vi "GUI.Config Test GENERICO.vi"() -> ()   [LabVIEW 2009]
panel:
  in  "QUIT 2":bool
  in  "QUIT":bool
  in  "default":bool
  in  "Limits Measurements ADC":string[][](table)
  in  "stop":bool
  in  "Lim offset Dig":cluster{"Max Dig":dbl}={"Max Dig"=0.05} {"Max Dig" format="%.3g"}
  in  "Lim Offset Analog":cluster{"Max Analog":dbl, "Min Analog":dbl}={"Max Analog"=0.05, "Min Analog"=-0.05} {"Min Analog" format="%.3g"; "Max Analog" format="%.3g"}
  in  "Vin Rate Adders":i32[](listbox)
  in  "Limits Rate Scan":cluster{"High":dbl[], "Low":dbl[]}={"High"=[0.15, 0.242, 0.331, 0.425, 0.512, 0.6, 0.688, 0.774, 0.847, 0.91], "Low"=[0.021, 0.11, 0.189, 0.27, 0.347, 0.421, 0.487, 0.551, 0.601, 0.635]} {"Low" format="%1.4f"; "High" format="%1.3f"}
  in  "Vin Rate Scan":i32[](listbox)
  in  "Limits Max PN Min NP":T1={"Max P inferior"=1.888, "Max P superior"=2.177000045776367, "Min N superior"=0.818, "Min N inferior"=0.73, "Max N superior"=1.475, "Max N inferior"=1.322, "Min P inferior "=1.321, "Min P superior"=1.474} {"Min P superior" format="%.3g"; "Min P inferior" format="%.3g"; "Max N inferior" format="%.3g"; "Max N superior" format="%.3g"; "Min N inferior" format="%.3g"; "Min N superior" format="%.3g"; "Max P superior" format="%.3g"; "Max P inferior" format="%.3g"}
  in  "Limits ADC":cluster{"Low":dbl[], "High":dbl[], "Vin":dbl[]}={"Low"=[1.9, 1.3, 0.65, 0.0, 1.6, 1.4, 1.4, 0.9, 2.1, 0.85, 1.9], "High"=[2.1, 1.5, 0.85, 0.1, 1.4, 1.2, 1.2, 0.7, 1.9, 0.65, 1.7], "Vin"=[1.9, 1.3, 0.65, 0.0, 1.6, 1.4, 1.4, 0.9, 2.1, 0.85, 1.9]} {"Vin" format="%1.3f"; "High" format="%1.4f"; "Low" format="%1.3f"}
  in  "Test ADC 2":cluster{"Repeats ADC":i32, "Max Desviation":dbl}={"Repeats ADC"=100, "Max Desviation"=0.1}
  in  "Tab Control":T2(tab)
  in  "Ruta Destino":path
  in  "Place":string(combo)
  in  "Operator's Name":string(combo)
  out "ASIC'S Number":string
  in  "Config Test offset Digital":bool
  in  "Config Test offset Analog":bool
  in  "Config Test Rate Scan Adders":bool
  in  "Config Test Rate Scan":bool
  in  "Config Test Max PN Min PN":bool
  in  "Config Test ADC":bool
  in  "Config Test Register":bool
  in  "Test offset Digital":bool
  in  "Test offset Analog":bool
  in  "Test Rate Scan Adders":bool
  in  "Test Rate Scan":bool
  in  "Test Max PN Min PN":bool
  in  "Test ADC":bool
  in  "Test Register":bool
  in  "Enum":enum16{""}(ring)
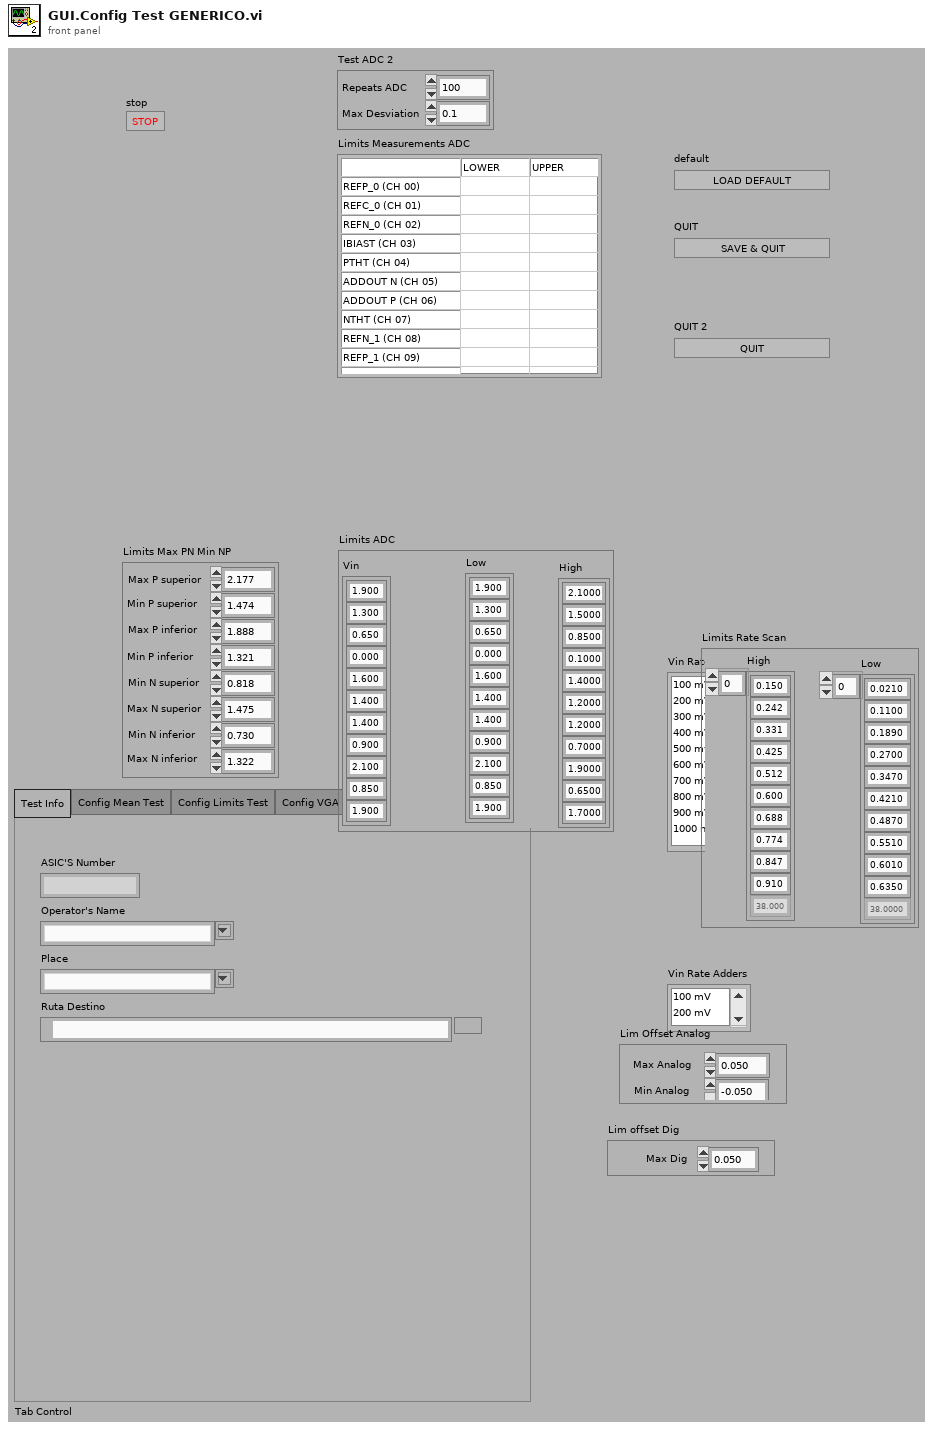
[diagram p1: front panel]
types:
  T1 = cluster{"Max P inferior":dbl, "Max P superior":dbl, "Min N superior":dbl, "Min N inferior":dbl, "Max N superior":dbl, "Max N inferior":dbl, "Min P inferior ":dbl, "Min P superior":dbl}
  T2 = enum32{"Test Info", "Config Mean Test", "Config Limits Test", "Config VGA", "Config Hardware Test"}
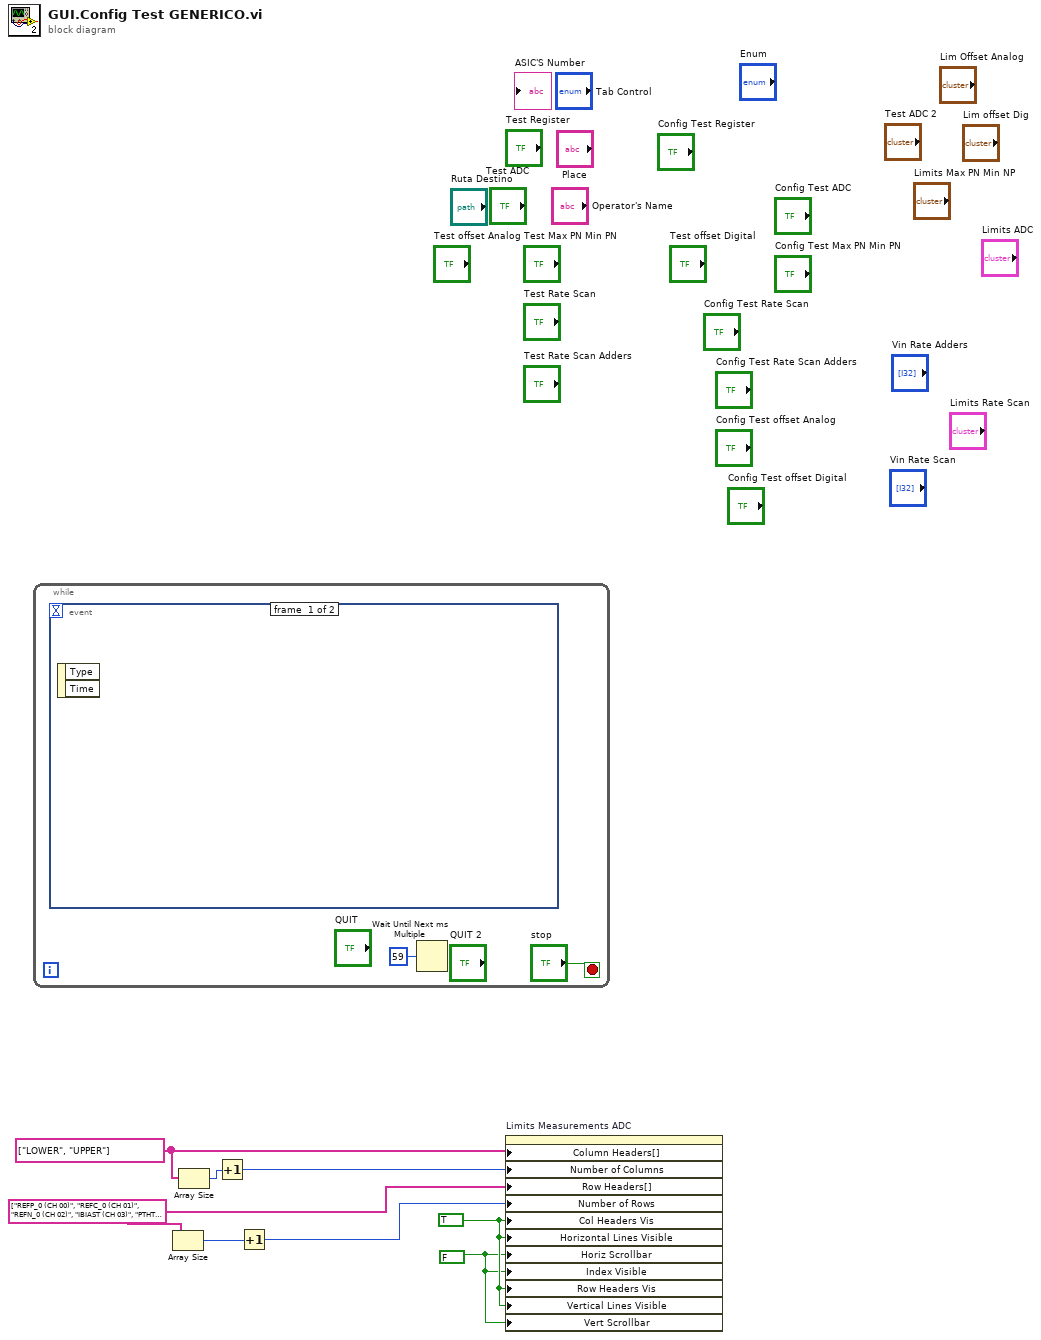
[diagram p0: block diagram]
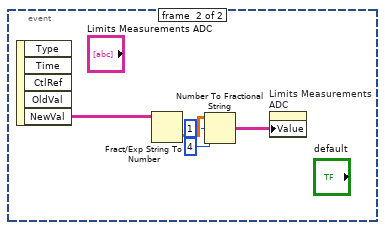
[diagram p2: hidden frame]
diagram:
  w1 = FALSE ("Autosizing Row Height")
  w2 = TRUE ("Autosizing Row Height")
  w8 = string[] ["LOWER", "UPPER"] ("Column Headers")
  w7 = string[] ["REFP_0 (CH 00)", "REFC_0 (CH 01)", "REFN_0 (CH 02)", "IBIAST (CH 03)", "PTHT (CH 04)", "ADDOUT N (CH 05)", "ADDOUT P (CH 06)", "NTHT (CH 07)", "REFN_1 (CH 08)", "REFP_1 (CH 09)", "VCOM (CH 10)"] ("Column Headers")
  n1 = while {
    stop <- "stop" stop-if-true
    n2 = event shown="[1] \"Limits Measurements ADC \": Value Change" {
      selector: _ -> [_ _]
      dyn-events: _ -> [_ _]
      timeout: _ -> [_ _]
      event #0 {
        n3 = event-data() -> ()  [unwired: 1 in, 2 out]
      }
      event #1 {
        n4 = event-data() -> ("NewVal"=w13:string[][])  [unwired: 1 in, 4 out]
        n5 = Fract/Exp String To Number(string=w13) -> (number=w15:dbl[][])  [unwired: 3 in, 1 out]
        n6 = Number To Fractional String(number=w15, width (-)=i16 1, precision (6)=i16 4) -> (F-format string=w14:string[][])  [unwired: 1 in]
        n7 = property on="Limits Measurements ADC" class="Tbl (strict)"("Value"=w14) -> ()  [unwired: 2 in, 2 out]
      }
    }
    n8 = Wait Until Next ms Multiple(millisecond multiple=u32 59) -> ()  [unwired: 1 out]
  }
  n9 = Array Size(array=w7) -> (size(s)=w5:i32)
  n10 = Array Size(array=w8) -> (size(s)=w6:i32)
  n11 = Increment(x=w6) -> (x+1=w4:i32)
  n12 = Increment(x=w5) -> (x+1=w3:i32)
  n13 = property on="Limits Measurements ADC" class="Table (strict)"("Column Headers[]"=w8, "Number of Columns"=w4, "Row Headers[]"=w7, "Number of Rows"=w3, "Col Headers Vis"=w2, "Horizontal Lines Visible"=w2, "Horiz Scrollbar"=w1, "Index Visible"=w1, "Row Headers Vis"=w2, "Vertical Lines Visible"=w2, "Vert Scrollbar"=w1) -> ()  [unwired: 2 in, 2 out]
